vi "action.vi"(0 "HGF_FGV_Append":refnum<class "HGF_FGV_Append.lvclass">, 2 "Objects":refnum<class>[](array[class]), 5 "error in (no error)":errorcluster) -> (14 "dup HGF_FGV_Append":refnum<class "HGF_FGV_Append.lvclass">, 16 "dup Objects":refnum<class>[](array[class]), 19 "error out":errorcluster)   [LabVIEW 2012, in "HGF_FGV.lvlib" / "HGF_FGV_Append.lvclass"]
doc: "Append object array."
uses:
  HGF_FGV_Append.lvclass
  HGF_FGV_Append.lvclass/HGF_FGV_Append.ctl
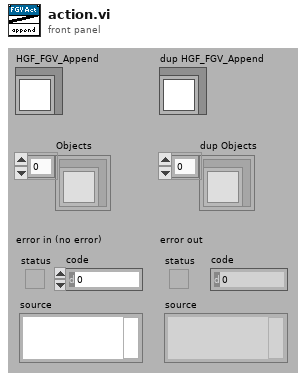
[diagram p1: front panel]
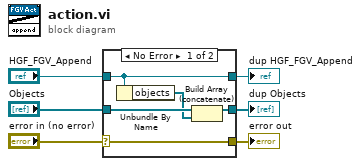
[diagram p0: block diagram]
diagram:
  n1 = case shown="No Error" "error in (no error)" {
    selector: "error in (no error)" -> [w11 w14]
    tunnel: [w11 w14] -> w5
    tunnel: [w10 w13] -> w3
    tunnel: "HGF_FGV_Append" -> [w10 w13]
    tunnel: [w8 w12] -> w2
    tunnel: "Objects" -> [w9 w12]
    frame No Error {
      n2 = Unbundle By Name(w10) -> ("objects"=w7:refnum<class>[])
      n3 = Build Array (concatenate)(w9, w7) -> (w8:refnum<class>[])
    }
    frame Error {
    }
  }
  "error out" <- w5
  "dup HGF_FGV_Append" <- w3
  "dup Objects" <- w2
